vi "Post-Processing VI Bin Files.vi"() -> ()   [LabVIEW 2014]
uses:
  <vilib>/Utility/config.llb/Read Key (I32).vi
  <vilib>/Utility/config.llb/Read Key (Double).vi
  <vilib>/Utility/config.llb/NI_LVConfig.lvlib
panel:
  out "Range":dbl
  out "Bits":dbl
  out "Points Per A Scan":i32
  out "A-Scans Per BScan":i32
  in  "Min / Max in dB (Contrast)":cluster{dbl, dbl}(slide)={-13.295819935691327, 5.096463022508033} scale=-40.0..60.0
  in  "Create 3D Data":bool=TRUE
  in  "Max":sgl format="%0.2f"
  in  "Min":sgl format="%0.2f"
  out "Binary File Handle":refnum<file>
  in  "Create En Face Software Event":bool=TRUE
  out "En Face":sgl[][](graph)
  out "error out":errorcluster
  in  "En Face Upper Depth":i32=60
  in  "En Face Lower Depth":i32=300
  in  "B-Scan Select":i32(slide) scale=0.0..500.0
  out "BScan":u8[][](graph)
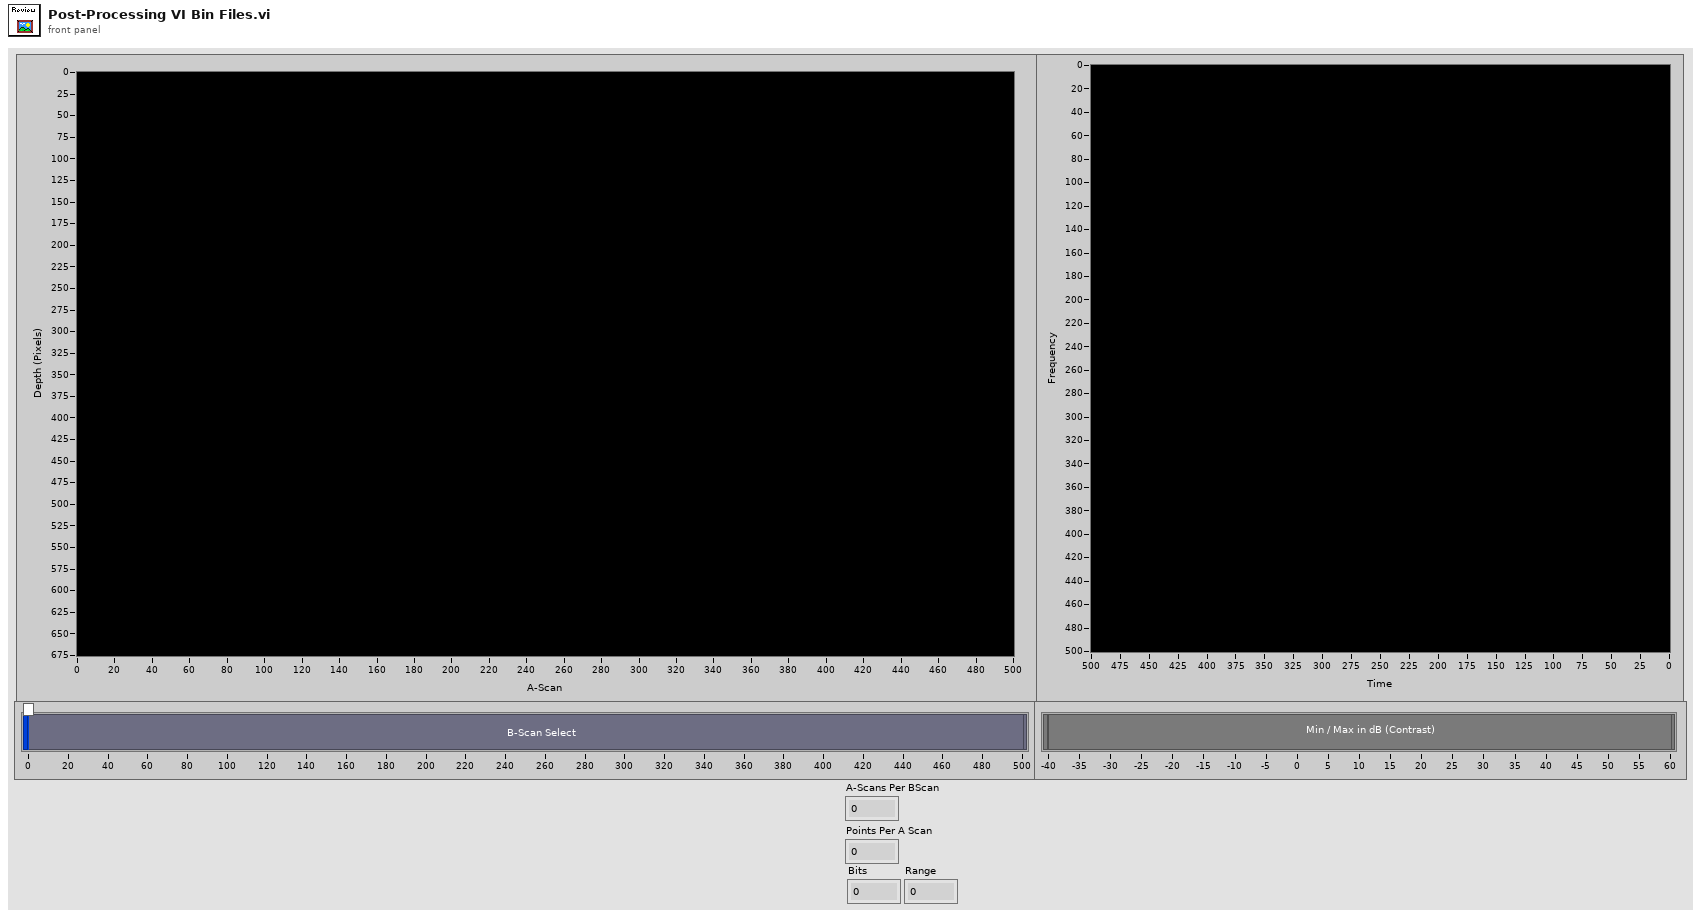
[diagram p1: front panel]
types:
  T1 = typedef "NI_LVConfig.lvlib/Config Data RefNum.ctl" = refnum<k1>
  T2 = typedef "imagedata.ctl" = cluster{"image type":i32, "image depth":i32, "image":u8[], "mask":u8[], "colors":u32[], "Rectangle":cluster{"left":i16, "top":i16, "right":i16, "bottom":i16}}
  T3 = typedef "LVCursorListTypeDef.ctl" = cluster{"Name":string, "Color":u32, "Style":u8, "Point Style":u8, "Name Visible":bool, "Allow Drag":bool, "Cursor Mode":u32, "Plot":i32, "Index":i32, "Position":cluster{"X":dbl, "Y":dbl}, "X Scale":u32, "Y Scale":u32, "Watch Plots":i32[], "Watch All Plots":bool, "Plot Area":i32, "Label Offset":cluster{"X":dbl, "Y":dbl}}[]
  T4 = cluster{"Name":string, "Color":u32, "Style":u8, "Point Style":u8, "Name Visible":bool, "Allow Drag":bool, "Cursor Mode":u32, "Plot":i32, "Index":i32, "Position":cluster{"X":dbl, "Y":dbl}, "X Scale":u32, "Y Scale":u32, "Watch Plots":i32[], "Watch All Plots":bool, "Plot Area":i32, "Label Offset":cluster{"X":dbl, "Y":dbl}}
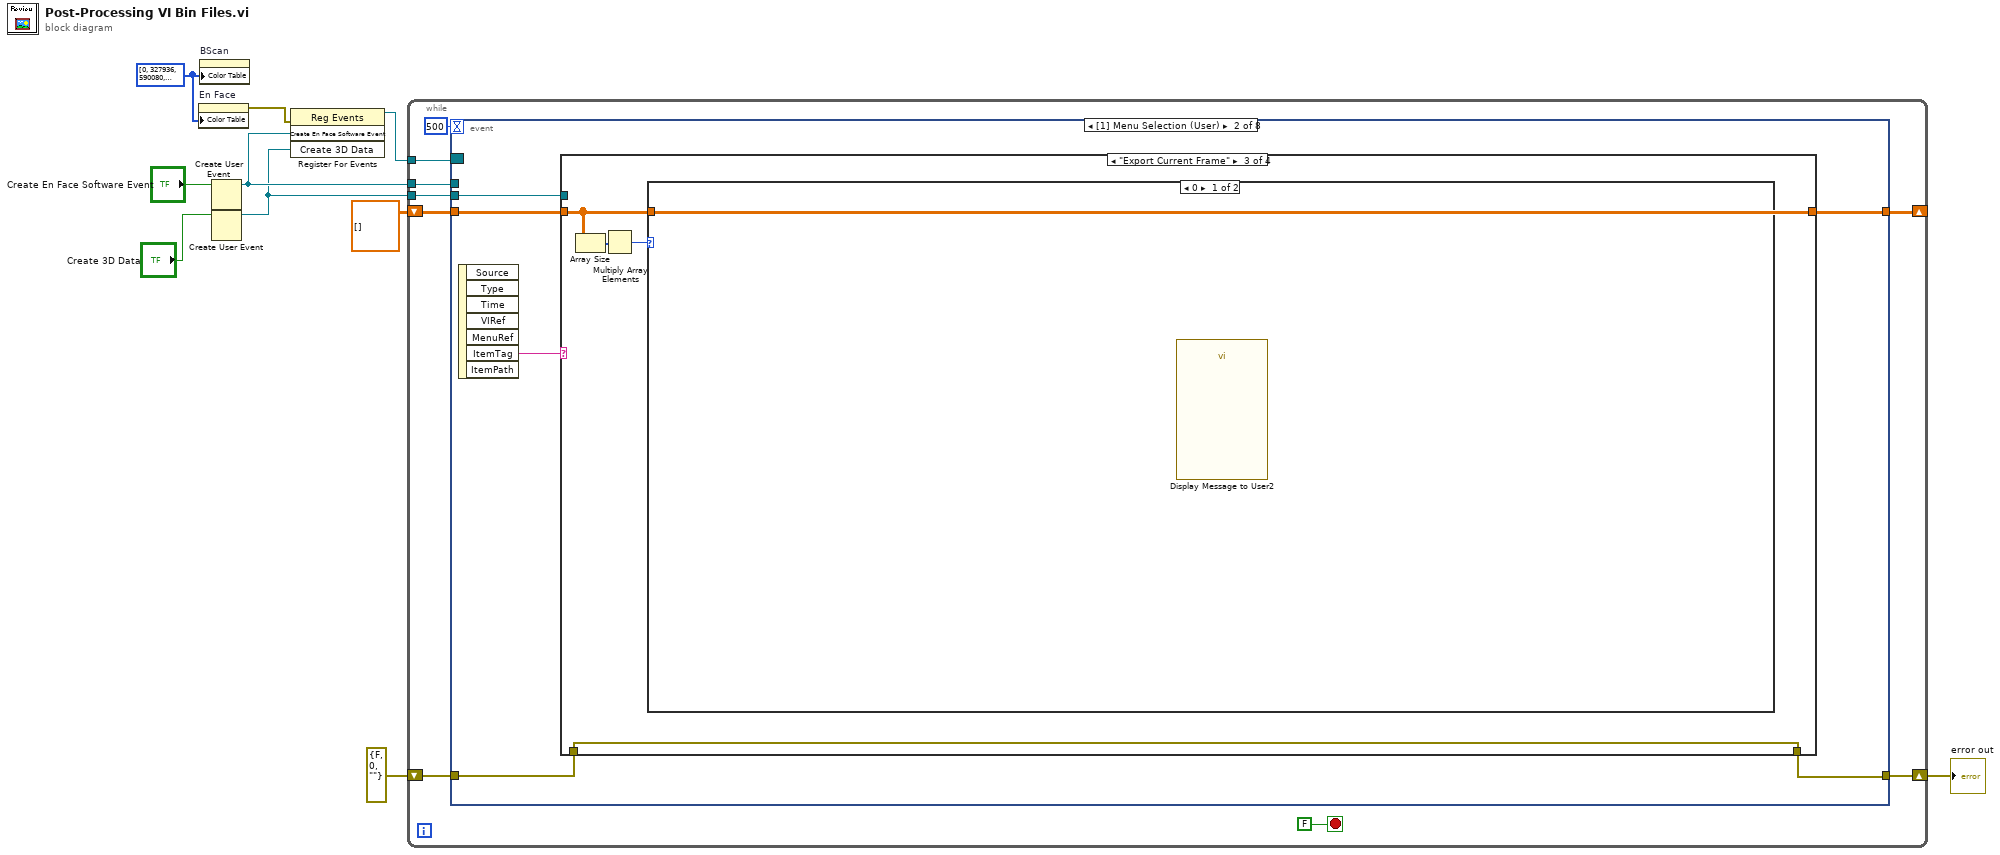
[diagram p0: block diagram]
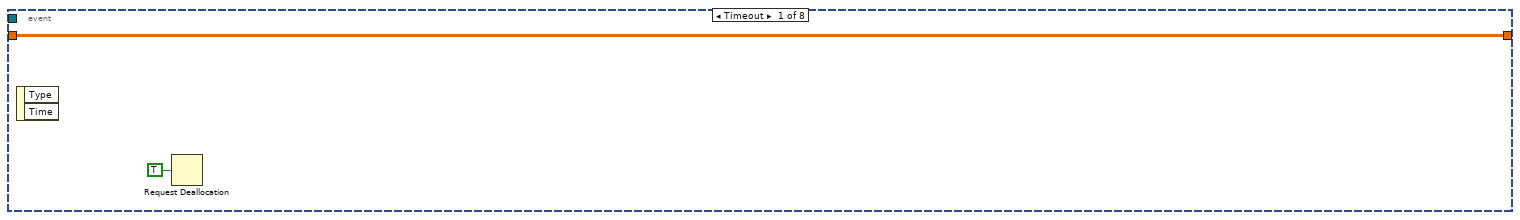
[diagram p2: hidden frame]
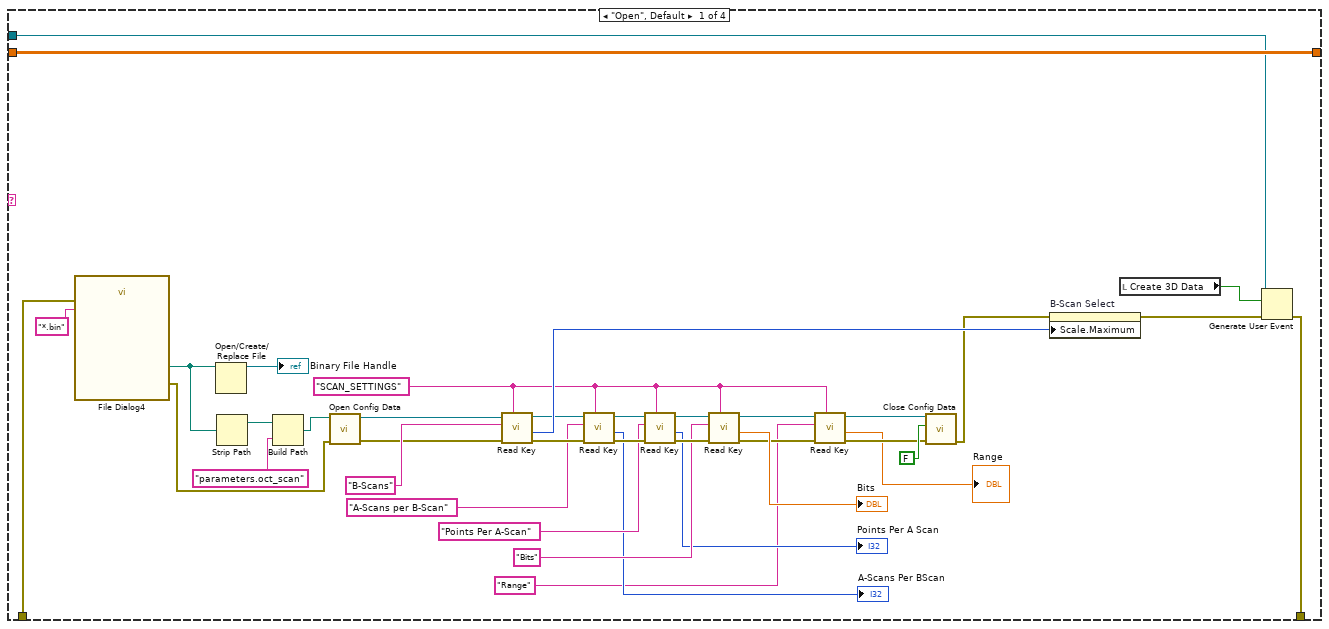
[diagram p3: hidden frame]
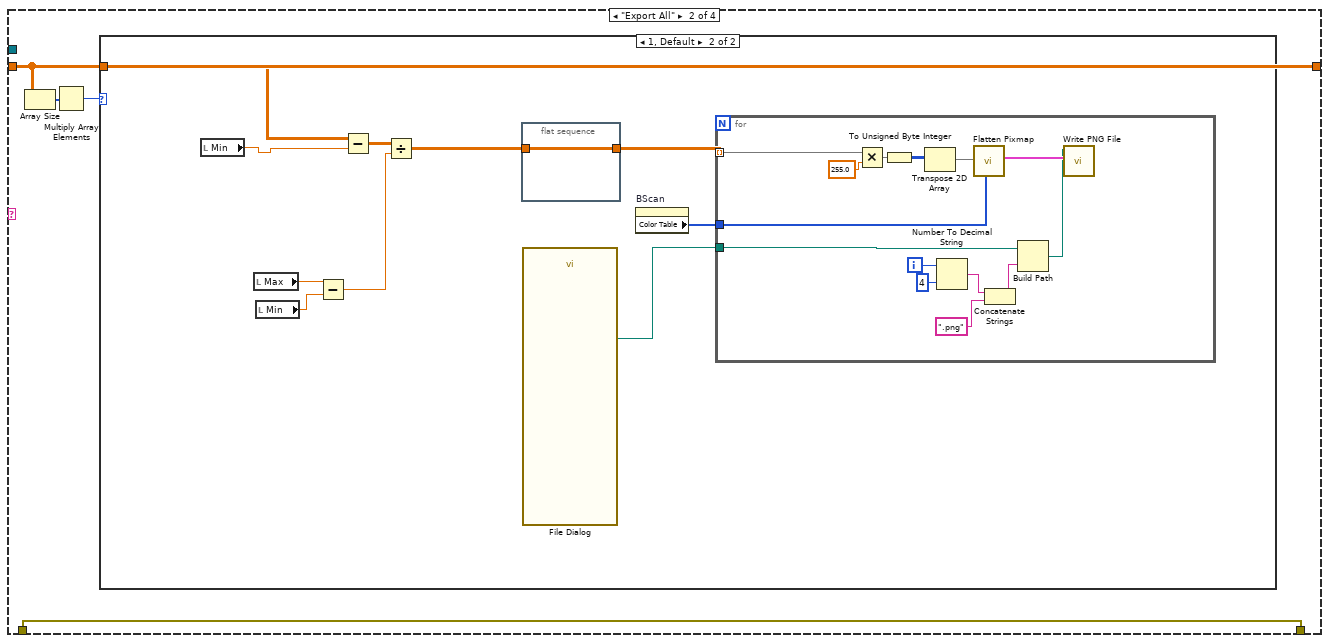
[diagram p4: hidden frame]
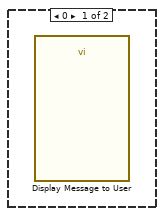
[diagram p5: hidden frame]
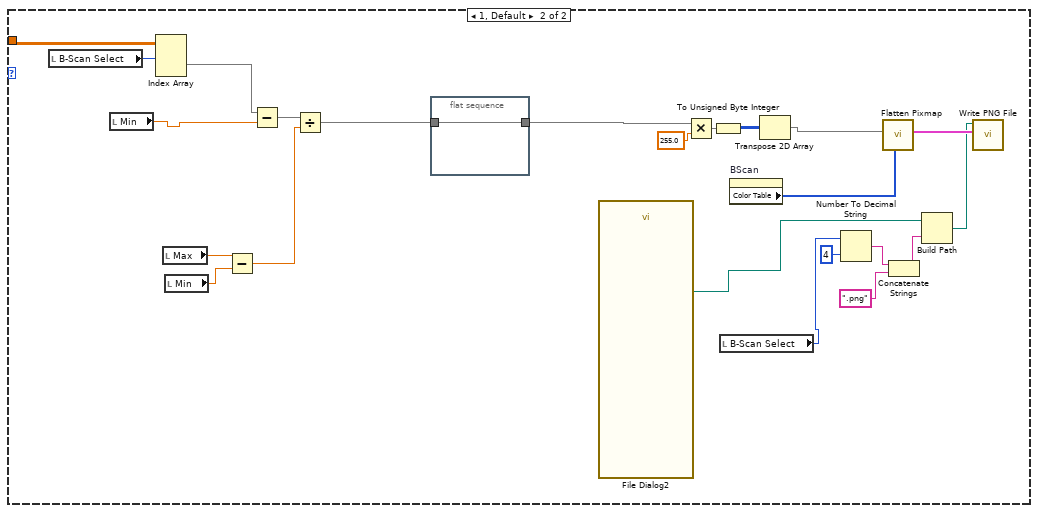
[diagram p6: hidden frame]
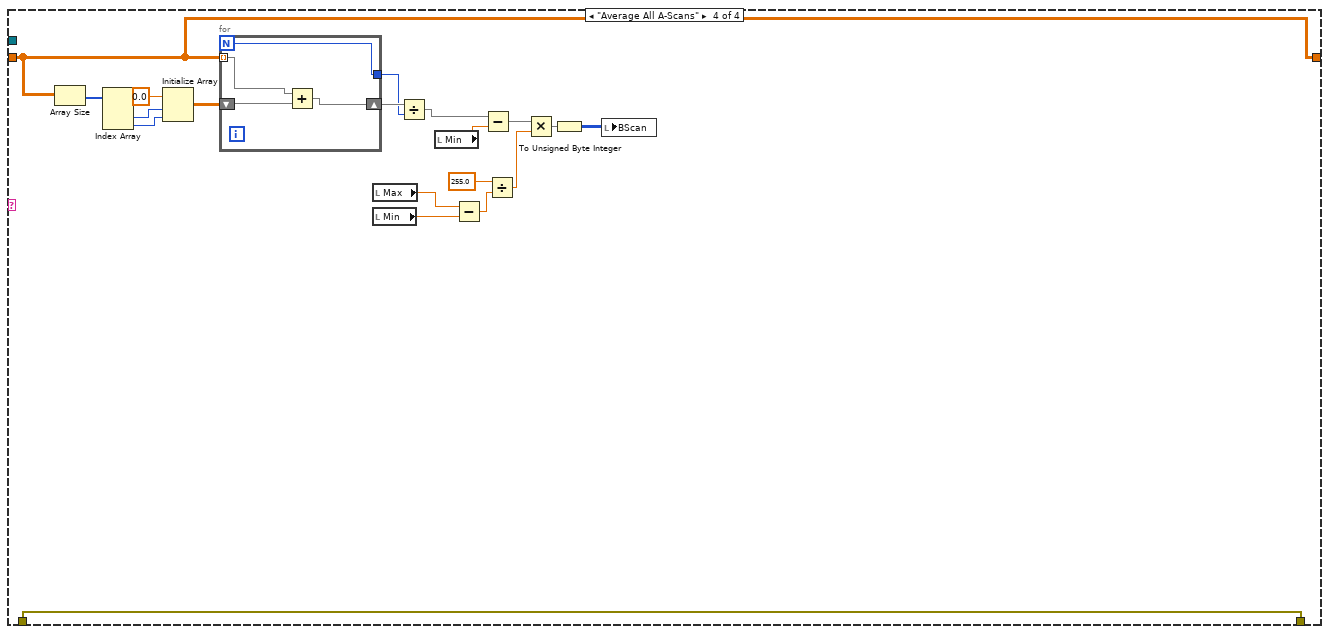
[diagram p7: hidden frame]
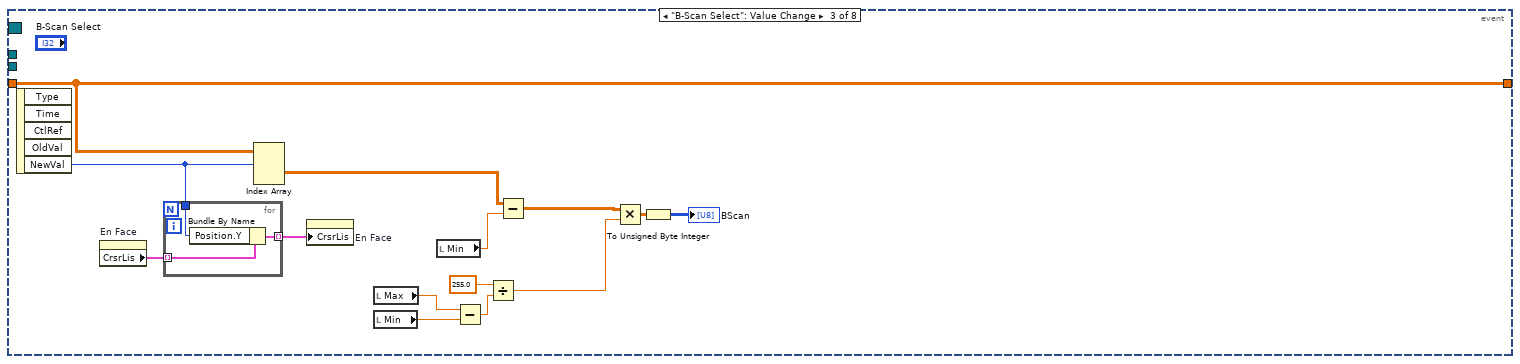
[diagram p8: hidden frame]
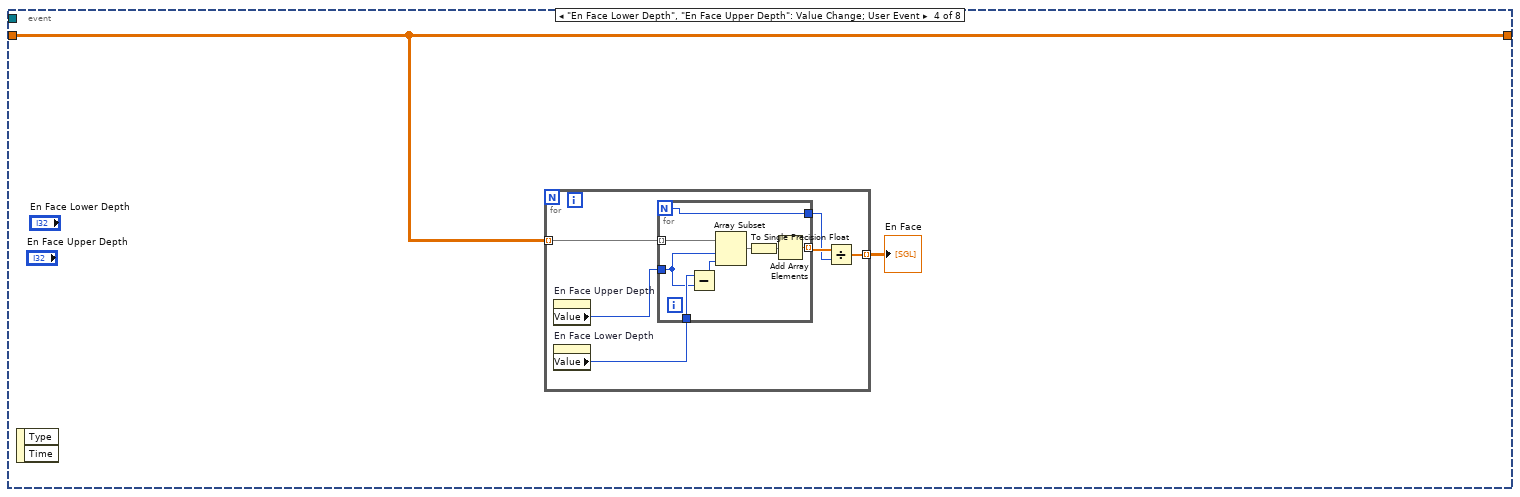
[diagram p9: hidden frame]
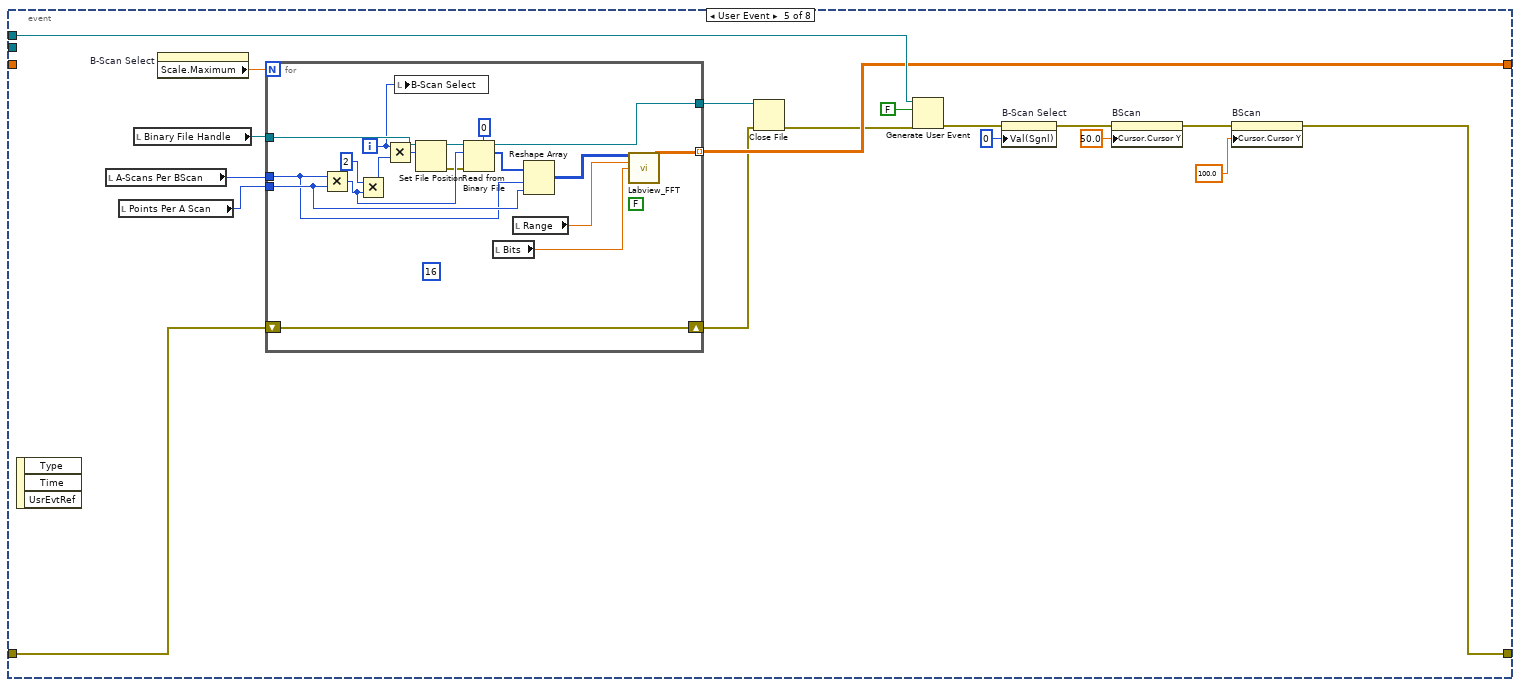
[diagram p10: hidden frame]
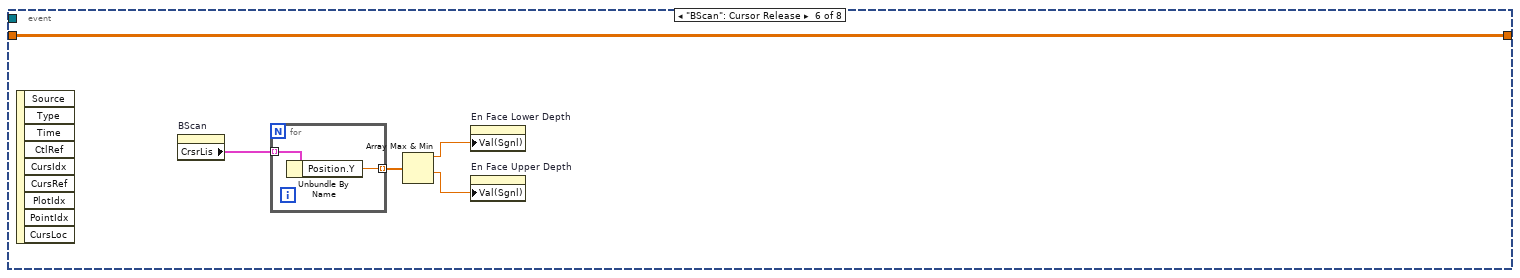
[diagram p11: hidden frame]
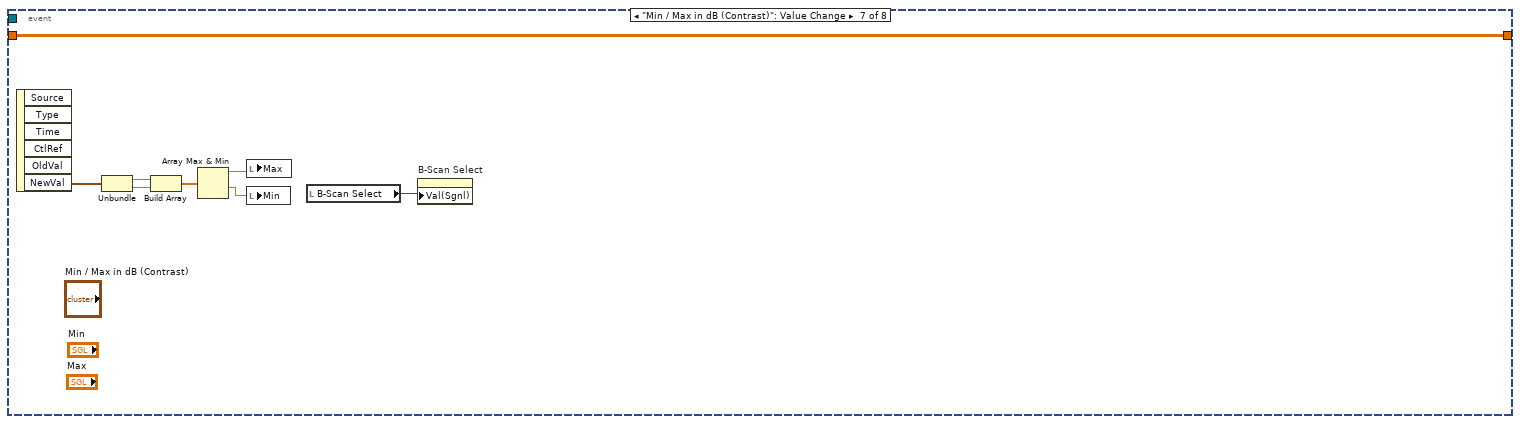
[diagram p12: hidden frame]
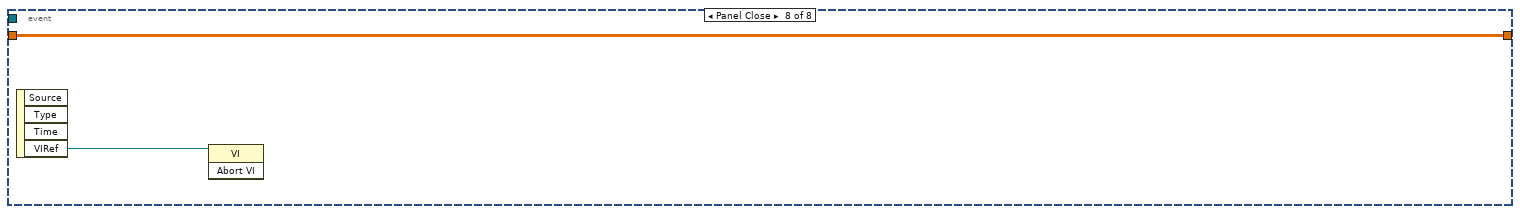
[diagram p13: hidden frame]
diagram:
  w3 = u32[] [0, 327936, 590080, 852224, 983296, 1114624, 1180160, 1311232, 1442304, 1573632, 1704704, 1770240, 1901312, 1966848, 2098176, 2163712, 2294784, 2491392, 2557184, 2688256, 2753792, 2884864, 2950656, 3081728, 3147264, 3344129, 3475457, 3540993, 3672321, 3738113, 3869185, 3934977, 4066305, 4197633, 4328961, 4394497, 4460289, 4591617, 4657409, 4788481, 4854273, 4985601, 5116929, 5248257, 5314049, 5379841, 5511169, 5576961, 5708033, 5773825, 5905153, 6036482, 6167810, 6233346, 6299138, 6430466, 6496258, 6562050, 6693634, 6759426, 6890754, 7022082, 7087874, 7153666, 7284994, 7350786, 7482114, 7547906, 7613698, 7745026, 7876354, 8007682, 8073474, 8139522, 8205314, 8336642, 8467970, 8533763, 8599555, 8665347, 8731139, 8862467, 8993795, 9059587, 9125380, 9191428, 9257220, 9388548, 9454340, 9520132, 9585924, 9717253, 9848837, 9914629, 9980165, 10045957, 10177541, 10243334, 10309126, 10375174, 10440966, 10572294, 10703623, 10769416, 10835208, 10901256, 10967049, 11033097, 11033609, 11099401, 11165450, 11231242, 11231754, 11297547, 11363339, 11429131, 11495180, 11495692, 11561740, 11693069, 11758861, 11759373, 11825165, 11891214, 11957006, 12022799, 12023311, 12089103, 12220944, 12286736, 12286736, 12352529, 12418577, 12484370, 12550162, 12615954, 12681747, 12747796, 12813588, 12813845, 12879894, 12945686, 13077015, 13142808, 13143064, 13208856, 13274905, 13340697, 13340953, 13472282, 13538075, 13604379, 13670172, 13735964, 13801757, 13867550, 13933343, 13999392, 13999648, 14065441, 14131234, 14197027, 14197541, 14263334, 14329383, 14395176, 14460969, 14592553, 14658346, 14724139, 14789932, 14790189, 14856238, 14922287, 14988080, 15053873, 15054130, 15119923, 15185972, 15251765, 15317559, 15383353, 15449146, 15449660, 15515454, 15515968, 15516226, 15582021, 15582278, 15582536, 15648587, 15648844, 15714639, 15714897, 15715155, 15780949, 15781463, 15847256, 15847770, 15848028, 15913823, 15914081, 15979875, 15980133, 15980391, 16046441, 16046444, 16046703, 16046705, 16112500, 16113015, 16113274, 16113277, 16179072, 16179330, 16179588, 16245384, 16245387, 16245389, 16245648, 16311443, 16376982, 16377241, 16377499, 16443294, 16443553, 16443555, 16443815, 16509866, 16510124, 16510127, 16575923, 16575924, 16576182, 16576441, 16576443, 16576702, 16576705, 16576963, 16577222, 16577224, 16577482, 16577485, 16577743, 16577745, 16578004, 16578262, 16578264, 16578523, 16578782, 16579040, 16579299, 16579301, 16579303, 16579562, 16579821] ("Color Table")
  n1 = property on="En Face" class="IntGraph (strict)"("Color Table"=w3) -> (error out=w2:errorcluster)  [unwired: 2 in, 1 out]
  n2 = property on="BScan" class="IntGraph (strict)"("Color Table"=w3) -> ()  [unwired: 2 in, 2 out]
  n3 = Create User Event(user event datatype="Create En Face Software Event") -> (user event=w9:refnum<user-event>)  [unwired: 1 in, 1 out]
  n4 = Create User Event(user event datatype="Create 3D Data") -> (user event=w8:refnum<user-event>)  [unwired: 1 in, 1 out]
  n5 = register-events(error in=w2, w9, w8) -> (reference out=w10:refnum<event-registration>)  [unwired: 1 in, 1 out]
  n6 = while {
    tunnel: w10 -> [w17]
    tunnel: w9 -> [w16]
    tunnel: w8 -> [w15]
    shift-right: [w13] -> w4
    shift-left: errorcluster {"status"=FALSE, "code"=0, "source"=""} ("error constant") -> [w14]
    shift-right: [w11] -> _
    shift-left: sgl[][][] [] ("Int B-Scan Channel A") -> [w12]
    stop <- FALSE stop-if-true
    n7 = event shown="[1] Menu Selection (User)" {
      selector: w17 -> [_ _ _ _ _ _ _ _]
      dyn-events: _ -> [_ _ _ _ _ _ _ _]
      timeout: 500 -> [_ _ _ _ _ _ _ _]
      tunnel: w15 -> [_ w24 _ _ _ _ _ _]
      tunnel: w16 -> [_ _ _ _ w193 _ _ _]
      tunnel: w14 -> [_ w23 _ _ w192 _ _ _]
      tunnel: [_ w22 _ _ w181 _ _ _] -> w13
      tunnel: w12 -> [w21 w26 w146 w163 _ w215 w222 w230]
      tunnel: [w21 w25 w146 w163 w189 w215 w222 w230] -> w11
      event Timeout {
        n8 = event-data() -> ()  [unwired: 1 in, 2 out]
        n9 = Request Deallocation(TRUE ("flag")) -> ()
      }
      event Menu Selection (User) {
        n10 = event-data() -> ("ItemTag"=w27:string)  [unwired: 1 in, 6 out]
        n11 = case shown="\"Export Current Frame\"" w27 {
          tunnel: w26 -> [w65 w68 w97 w137]
          tunnel: [w65 w68 w97 w137] -> w25
          tunnel: w24 -> [w61 _ _ _]
          tunnel: w23 -> [w38 w69 w98 w141]
          tunnel: [w60 w69 w98 w141] -> w22
          frame "Open", Default {
            w32 = "SCAN_SETTINGS" ("section")
            n12 = call "File Dialog4"("error in"=w38, "pattern (all files)"="*.bin") -> ("selected path"=w58:path, "error out"=w40:errorcluster)  [unwired: 10 in, 2 out]
            n13 = Open/Create/Replace File(file path (use dialog)=w58) -> (refnum out=→"Binary File Handle":refnum<file>)  [unwired: 5 in, 2 out]
            n14 = Strip Path(path=w58) -> (stripped path=w57:path)  [unwired: 1 out]
            n15 = Build Path(base path=w57, name or relative path="parameters.oct_scan") -> (appended path=w55:path)
            n16 = call <vilib>:"Open Config Data.vi"("error in (no error)"=w40, "configuration file path"=w55) -> ("error out"=w53:errorcluster, "refnum"=w52:T1)  [unwired: 7 in, 1 out]
            n17 = call-poly <vilib>:"Read Key.vi"("section"=w32, "error in (no error)"=w53, "key"="B-Scans", "refnum"=w52) -> ("error out"=w49:errorcluster, "value"=w51:i32, "refnum out"=w48:T1)  [unwired: 4 in, 1 out]
            n18 = call-poly <vilib>:"Read Key.vi"("section"=w32, "error in (no error)"=w49, "key"="A-Scans per B-Scan", "refnum"=w48) -> ("error out"=w46:errorcluster, "value"=→"A-Scans Per BScan":i32, "refnum out"=w45:T1)  [unwired: 4 in, 1 out]
            n19 = call-poly <vilib>:"Read Key.vi"("section"=w32, "error in (no error)"=w46, "key"="Points Per A-Scan", "refnum"=w45) -> ("error out"=w43:errorcluster, "value"=→"Points Per A Scan":i32, "refnum out"=w42:T1)  [unwired: 4 in, 1 out]
            n20 = call-poly <vilib>:"Read Key.vi"("section"=w32, "error in (no error)"=w43, "key"="Bits", "refnum"=w42) -> ("error out"=w33:errorcluster, "value"=→"Bits":dbl, "refnum out"=w34:T1)  [unwired: 4 in, 1 out]
            n21 = call-poly <vilib>:"Read Key.vi"("section"=w32, "error in (no error)"=w33, "key"="Range", "refnum"=w34) -> ("error out"=w29:errorcluster, "value"=→"Range":dbl, "refnum out"=w30:T1)  [unwired: 4 in, 1 out]
            n22 = call <vilib>:"Close Config Data.vi"("error in (no error)"=w29, "write file if changed (T)"=FALSE, "refnum"=w30) -> ("error out"=w39:errorcluster)  [unwired: 7 in, 1 out]
            n23 = property on="B-Scan Select" class="Slide (strict)"(error in=w39, "Scale.Maximum"=w51) -> (error out=w63:errorcluster)  [unwired: 1 in, 1 out]
            n24 = local read "Create 3D Data"() -> (w62:bool)
            n25 = Generate User Event(user event=w61, event data cluster=w62, error in=w63) -> (error out=w60:errorcluster)  [unwired: 1 in, 1 out]
          }
          frame "Export All" {
            n26 = Array Size(array=w68) -> (size(s)=w67:i32[])
            n27 = Multiply Array Elements(1:w67) -> (0:w66:i32)
            n28 = case shown="1, Default" w66 {
              tunnel: w68 -> [_ w79]
              frame 0 {
                n29 = call "Display Message to User"() -> ()  [unwired: 10 in, 2 out]
              }
              frame 1, Default {
                n30 = local read "Min"() -> (w73:sgl)
                n31 = local read "Max"() -> (w72:sgl)
                n32 = local read "Min"() -> (w71:sgl)
                n33 = Subtract(x=w72, y=w71) -> (x-y=w77:sgl)
                n34 = Subtract(x=w79, y=w73) -> (x-y=w78:sgl[][][])
                n35 = Divide(x=w78, y=w77) -> (x/y=w76:sgl[][][])
                n36 = flat-sequence {
                  tunnel: [w94] -> w75
                  tunnel: w76 -> [w94]
                  frame #0 {
                  }
                }
                n37 = call "File Dialog"() -> ("selected path"=w74:path)  [unwired: 12 in, 3 out]
                n38 = property on="BScan" class="IntGraph (strict)"() -> ("Color Table"=w70:u32[])  [unwired: 2 in, 2 out]
                n39 = for {
                  tunnel: w75 -> [w93] mode=indexing
                  tunnel: w74 -> [w87]
                  tunnel: w70 -> [w80]
                  i -> [w90]
                  n40 = Multiply(x=w93, y=sgl 255.0) -> (x*y=w91:sgl[][])
                  n41 = To Unsigned Byte Integer(number=w91) -> (unsigned 8bit integer=w82:u8[][])
                  n42 = Transpose 2D Array(2D array=w82) -> (transposed array=w81:u8[][])
                  n43 = Number To Decimal String(number=w90, width (-)=i16 4) -> (decimal integer string=w85:string)
                  n44 = call <vilib>:"Flatten Pixmap.vi"("colors"=w80, "8-bit pixmap"=w81) -> ("image data"=w88:T2)  [unwired: 9 in]
                  n45 = Concatenate Strings(w85, ".png" ("string")) -> (w83:string)
                  n46 = Build Path(base path=w87, name or relative path=w83) -> (appended path=w86:path)
                  n47 = call <vilib>:"Write PNG File.vi"("image data"=w88, "path to PNG file"=w86) -> ()  [unwired: 8 in, 2 out]
                }
              }
            }
          }
          frame "Export Current Frame" {
            n48 = Array Size(array=w97) -> (size(s)=w96:i32[])
            n49 = Multiply Array Elements(1:w96) -> (0:w95:i32)
            n50 = case shown="0" w95 {
              tunnel: w97 -> [_ w104]
              frame 0 {
                n51 = call "Display Message to User2"() -> ()  [unwired: 10 in, 2 out]
              }
              frame 1, Default {
                n52 = local read "B-Scan Select"() -> (w105:i32)
                n53 = local read "Min"() -> (w116:sgl)
                n54 = Index Array(array=w104, index (dim 0)=w105) -> (element=w103:sgl[][])  [unwired: 2 in]
                n55 = local read "Max"() -> (w115:sgl)
                n56 = local read "Min"() -> (w114:sgl)
                n57 = Subtract(x=w115, y=w114) -> (x-y=w120:sgl)
                n58 = Subtract(x=w103, y=w116) -> (x-y=w121:sgl[][])
                n59 = Divide(x=w121, y=w120) -> (x/y=w119:sgl[][])
                n60 = flat-sequence {
                  tunnel: [w122] -> w118
                  tunnel: w119 -> [w122]
                  frame #0 {
                  }
                }
                n61 = call "File Dialog2"() -> ("selected path"=w117:path)  [unwired: 12 in, 3 out]
                n62 = Multiply(x=w118, y=sgl 255.0) -> (x*y=w112:sgl[][])
                n63 = To Unsigned Byte Integer(number=w112) -> (unsigned 8bit integer=w100:u8[][])
                n64 = local read "B-Scan Select"() -> (w102:i32)
                n65 = property on="BScan" class="IntGraph (strict)"() -> ("Color Table"=w101:u32[])  [unwired: 2 in, 2 out]
                n66 = Transpose 2D Array(2D array=w100) -> (transposed array=w99:u8[][])
                n67 = Number To Decimal String(number=w102, width (-)=i16 4) -> (decimal integer string=w108:string)
                n68 = call <vilib>:"Flatten Pixmap.vi"("colors"=w101, "8-bit pixmap"=w99) -> ("image data"=w110:T2)  [unwired: 9 in]
                n69 = Concatenate Strings(w108, ".png" ("string")) -> (w106:string)
                n70 = Build Path(base path=w117, name or relative path=w106) -> (appended path=w109:path)
                n71 = call <vilib>:"Write PNG File.vi"("image data"=w110, "path to PNG file"=w109) -> ()  [unwired: 8 in, 2 out]
              }
            }
          }
          frame "Average All A-Scans" {
            n72 = Array Size(array=w137) -> (size(s)=w140:i32[])
            n73 = Index Array(array=w140) -> (element #2=w124:i32, element #3=w123:i32)  [unwired: 3 in, 1 out]
            n74 = Initialize Array(sgl 0.0 ("element"), w124, w123) -> (w138:sgl[][])
            n75 = for {
              N -> [w142]
              tunnel: w137 -> [w144] mode=indexing
              shift-right: [w143] -> w136
              shift-left: w138 -> [w145]
              tunnel: [w142] -> w135
              n76 = Add(x=w144, y=w145) -> (x+y=w143:sgl[][])
            }
            n77 = local read "Max"() -> (w132:sgl)
            n78 = local read "Min"() -> (w131:sgl)
            n79 = Divide(x=w136, y=w135) -> (x/y=w125:sgl[][])
            n80 = local read "Min"() -> (w126:sgl)
            n81 = Subtract(x=w132, y=w131) -> (x-y=w130:sgl)
            n82 = Subtract(x=w125, y=w126) -> (x-y=w129:sgl[][])
            n83 = Divide(x=sgl 255.0, y=w130) -> (x/y=w128:sgl)
            n84 = Multiply(x=w129, y=w128) -> (x*y=w127:sgl[][])
            n85 = To Unsigned Byte Integer(number=w127) -> (unsigned 8bit integer=w134:u8[][])
            n86 = local write "BScan"(w134) -> ()
          }
        }
      }
      event "B-Scan Select": Value Change {
        n87 = event-data() -> ("NewVal"=w158:i32)  [unwired: 1 in, 4 out]
        n88 = property on="En Face" class="IntGraph (strict)"() -> ("CrsrLis"=w159:T3)  [unwired: 2 in, 2 out]
        n89 = for {
          tunnel: w159 -> [w162] mode=indexing
          tunnel: w158 -> [w161]
          tunnel: [w160] -> w157 mode=indexing
          n90 = Bundle By Name(cluster=w162, "Position.Y"=w161) -> (w160:T4)
        }
        n91 = Index Array(array=w146, index (dim 0)=w158) -> (element=w147:sgl[][])  [unwired: 2 in]
        n92 = property on="En Face" class="IntGraph (strict)"("CrsrLis"=w157) -> ()  [unwired: 2 in, 2 out]
        n93 = local read "Max"() -> (w155:sgl)
        n94 = local read "Min"() -> (w154:sgl)
        n95 = local read "Min"() -> (w149:sgl)
        n96 = Subtract(x=w155, y=w154) -> (x-y=w153:sgl)
        n97 = Divide(x=sgl 255.0, y=w153) -> (x/y=w151:sgl)
        n98 = Subtract(x=w147, y=w149) -> (x-y=w152:sgl[][])
        n99 = Multiply(x=w152, y=w151) -> (x*y=w150:sgl[][])
        n100 = To Unsigned Byte Integer(number=w150) -> (unsigned 8bit integer=→"BScan":u8[][])
      }
      event "En Face Lower Depth", "En Face Upper Depth": Value Change; User Event {
        n101 = event-data() -> ()  [unwired: 1 in, 2 out]
        n102 = for {
          tunnel: [w165] -> w164 mode=indexing
          tunnel: w163 -> [w166] mode=indexing
          n103 = property on="En Face Upper Depth" class="DigNum (strict)"() -> ("Value"=w170:i32)  [unwired: 2 in, 2 out]
          n104 = property on="En Face Lower Depth" class="DigNum (strict)"() -> ("Value"=w169:i32)  [unwired: 2 in, 2 out]
          n105 = for {
            N -> [w175]
            tunnel: w166 -> [w178] mode=indexing
            tunnel: w170 -> [w171]
            tunnel: w169 -> [w172]
            tunnel: [w176] -> w168 mode=indexing
            tunnel: [w175] -> w167
            n106 = Subtract(x=w172, y=w171) -> (x-y=w173:i32)
            n107 = Array Subset(array=w178, index=w171, length=w173) -> (w177:sgl[])
            n108 = To Single Precision Float(number=w177) -> (single precision float=w174:sgl[])
            n109 = Add Array Elements(numeric array=w174) -> (sum=w176:sgl)
          }
          n110 = Divide(x=w168, y=w167) -> (x/y=w165:sgl[])
        }
        "En Face" <- w164
      }
      event User Event {
        n111 = event-data() -> ()  [unwired: 1 in, 3 out]
        n112 = local read "A-Scans Per BScan"() -> (w184:i32)
        n113 = local read "Points Per A Scan"() -> (w185:i32)
        n114 = local read "Binary File Handle"() -> (w195:refnum<file>)
        n115 = property on="B-Scan Select" class="Slide (strict)"() -> ("Scale.Maximum"=w194:dbl)  [unwired: 2 in, 2 out]
        n116 = for {
          N: w194 -> [_]
          tunnel: w195 -> [w211]
          tunnel: [w203] -> w189 mode=indexing
          tunnel: w184 -> [w200]
          tunnel: w185 -> [w201]
          shift-right: [w205] -> w187
          shift-left: w192 -> [w205]
          tunnel: [w204] -> w188
          i -> [w206]
          (unwired) FALSE ("Linear?")
          (unwired) u16 16 ("Card Resolution (bits)")
          n117 = Multiply(x=w200, y=w201) -> (x*y=w208:i32)
          n118 = Multiply(x=u32 2 ("y"), y=w208) -> (x*y=w210:u32)
          n119 = Multiply(x=w206, y=w210) -> (x*y=w212:u32)
          n120 = local write "B-Scan Select"(w206) -> ()
          n121 = Set File Position(offset (in bytes) (0)=w212, refnum=w211) -> (refnum out=w213:refnum<file>, error out=w207:errorcluster)  [unwired: 2 in]
          n122 = Read from Binary File(5:u16 0 ("width (-)"), 8:w207, 10:w208, 11:w213) -> (2:w202:u16[], 3:w204:refnum<file>)  [unwired: 2 in, 2 out]
          n123 = local read "Bits"() -> (w198:dbl)
          n124 = local read "Range"() -> (w197:dbl)
          n125 = Reshape Array(w202, w200, w201) -> (w199:u16[][])
          n126 = call "Labview_FFT.vi"("Channel A"=w199, "Range"=w197, "Bits"=w198) -> ("Int B-Scan Channel A"=w203:sgl[][])  [unwired: 12 in]
        }
        n127 = Close File(refnum=w188, error in=w187) -> (error out=w186:errorcluster)  [unwired: 1 out]
        n128 = Generate User Event(user event=w193, event data cluster=FALSE ("event data"), error in=w186) -> (error out=w191:errorcluster)  [unwired: 1 in, 1 out]
        n129 = property on="B-Scan Select" class="Slide (strict)"(error in=w191, "Val(Sgnl)"=0 ("Value (Signaling)")) -> (error out=w183:errorcluster)  [unwired: 1 in, 1 out]
        n130 = property on="BScan" class="IntGraph (strict)"(error in=w183, "Cursor.Cursor Y"=50.0 ("Cursor.Cursor Position:Cursor Y")) -> (error out=w182:errorcluster)  [unwired: 1 in, 1 out]
        n131 = property on="BScan" class="IntGraph (strict)"(error in=w182, "Cursor.Cursor Y"=100.0 ("Cursor.Cursor Position:Cursor Y")) -> (error out=w181:errorcluster)  [unwired: 1 in, 1 out]
      }
      event "BScan": Cursor Release {
        n132 = event-data() -> ()  [unwired: 1 in, 9 out]
        n133 = property on="BScan" class="IntGraph (strict)"() -> ("CrsrLis"=w219:T3)  [unwired: 2 in, 2 out]
        n134 = for {
          tunnel: w219 -> [w221] mode=indexing
          tunnel: [w220] -> w218 mode=indexing
          n135 = Unbundle By Name(w221) -> ("Position.Y"=w220:dbl)
        }
        n136 = Array Max & Min(array=w218) -> (max value=w216:dbl, min value=w217:dbl)  [unwired: 2 out]
        n137 = property on="En Face Lower Depth" class="DigNum (strict)"("Val(Sgnl)"=w216) -> ()  [unwired: 2 in, 2 out]
        n138 = property on="En Face Upper Depth" class="DigNum (strict)"("Val(Sgnl)"=w217) -> ()  [unwired: 2 in, 2 out]
      }
      event "Min / Max in dB (Contrast)": Value Change {
        n139 = event-data() -> ("NewVal"=w229:cluster{dbl, dbl})  [unwired: 1 in, 5 out]
        n140 = Unbundle(w229) -> (w227:dbl, w228:dbl)
        n141 = Build Array(w227, w228) -> (w226:dbl[])
        n142 = Array Max & Min(array=w226) -> (max value=w224:dbl, min value=w225:dbl)  [unwired: 2 out]
        n143 = local write "Max"(w224) -> ()
        n144 = local write "Min"(w225) -> ()
        n145 = local read "B-Scan Select"() -> (w223:i32)
        n146 = property on="B-Scan Select" class="Slide (strict)"("Val(Sgnl)"=w223) -> ()  [unwired: 2 in, 2 out]
      }
      event Panel Close {
        n147 = event-data() -> ("VIRef"=w231:refnum<vi>)  [unwired: 1 in, 3 out]
        n148 = invoke class="VI" method="Abort VI"(reference=w231) -> ()  [unwired: 2 in, 3 out]
      }
    }
  }
  "error out" <- w4
